vi "Configure Joystick Axis Translation.vi"(5 "Speed Profile (0: no change)":u16(ring) items=["no change", "linear", "squared", "cubed"], 6 "Axis Direction (0: no change)":u16(ring) items=["no change", "default direction", "inverted"], 7 "Maximum Speed (0)":u32, 8 "error in (no error)":errorcluster, 9 "Joystick Device Number":string, 10 "Joystick Axis Number (1)":i32=1 min=1 step=1, 11 "VISA resource name":refnum<visa-resource-name>) -> (0 "error out":errorcluster, 3 "VISA resource name out":refnum<visa-resource-name>)   [LabVIEW 2015, in "Zaber A Series.lvlib"]
doc: "Use this VI to configure the control behavior of one axis of a joystick device. \n\nEnter the device number of the joystick to be configured and select an axis to configure - 1 is the horizontal axis, 2 the vertical, and 3 is the rotation of the knob on the end of the stick. \n\nThe Maximum Speed input sets the highest velocity that will be sent to the axis the joystick controls.\n\nThe Speed Profile input controls the curve by which joystick positions are translated into velocity data.\n\nThe Axis Direction input controls whether positive joystick deflection becomes positive or negative velocity.\n\nThis VI requires that the serial port has already been opened."
uses:
  Zaber A Series.lvlib
  Private/All Commands.ctl
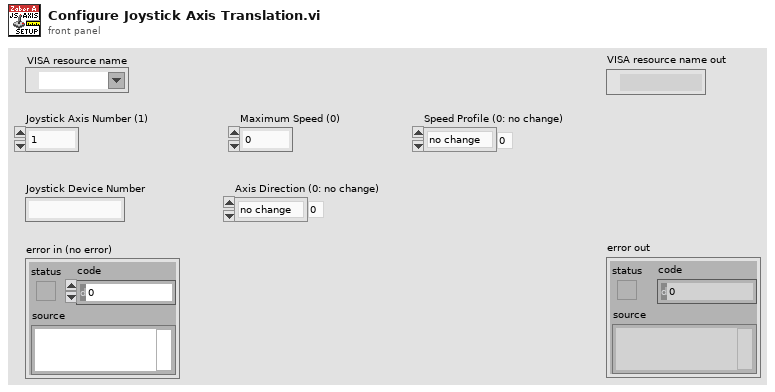
[diagram p1: front panel]
types:
  T1 = typedef "Zaber A Series.lvlib/All Commands.ctl" = string
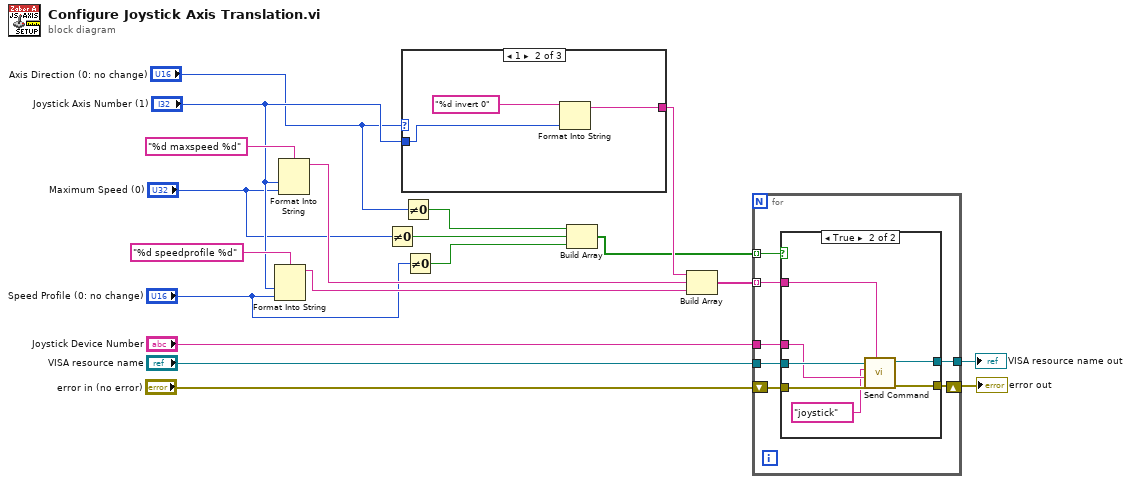
[diagram p0: block diagram]
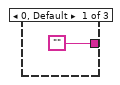
[diagram p3: hidden frame]
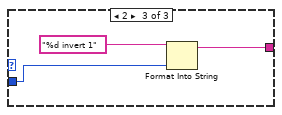
[diagram p4: hidden frame]
diagram:
  n1 = Format Into String(format string="%d speedprofile %d", "Joystick Axis Number (1)", "Speed Profile (0: no change)") -> (resulting string=w13:string)  [unwired: 2 in, 1 out]
  n2 = Format Into String(format string="%d maxspeed %d", "Joystick Axis Number (1)", "Maximum Speed (0)") -> (resulting string=w9:string)  [unwired: 2 in, 1 out]
  n3 = Not Equal To 0?(x="Maximum Speed (0)") -> (x != 0?=w11:bool)
  n4 = case shown="1" "Axis Direction (0: no change)" {
    tunnel: ["" w22 w25] -> w14
    tunnel: "Joystick Axis Number (1)" -> [_ w21 w24]
    frame 0, Default {
    }
    frame 1 {
      n5 = Format Into String(format string="%d invert 0", w21) -> (resulting string=w22:string)  [unwired: 2 in, 1 out]
    }
    frame 2 {
      n6 = Format Into String(format string="%d invert 1", w24) -> (resulting string=w25:string)  [unwired: 2 in, 1 out]
    }
  }
  n7 = Not Equal To 0?(x="Axis Direction (0: no change)") -> (x != 0?=w10:bool)
  n8 = Not Equal To 0?(x="Speed Profile (0: no change)") -> (x != 0?=w15:bool)
  n9 = Build Array(w10, w11, w15) -> (w5:bool[])
  n10 = Build Array(w14, w9, w13) -> (w4:string[])
  n11 = for {
    tunnel: [w33] -> w17
    tunnel: w5 -> [w31] mode=indexing
    tunnel: w4 -> [w30] mode=indexing
    tunnel: "VISA resource name" -> [w29]
    tunnel: "Joystick Device Number" -> [w27]
    shift-right: [w32] -> w16
    shift-left: "error in (no error)" -> [w28]
    n12 = case shown="True" w31 {
      tunnel: [w35 w42] -> w33
      tunnel: [w34 w41] -> w32
      tunnel: w30 -> [_ w40]
      tunnel: w29 -> [w35 w39]
      tunnel: w28 -> [w34 w38]
      tunnel: w27 -> [_ w37]
      frame False {
      }
      frame True {
        n13 = call "Send Command.vi"("Data"=w40, "error in (no error)"=w38, "Device and Axis"=w37, "Command"=T1 "joystick" ("Complete Command List"), "VISA resource name"=w39) -> ("error out"=w41:errorcluster, "VISA resource name out"=w42:refnum<visa-resource-name>)  [unwired: 1 in, 4 out]
      }
    }
  }
  "VISA resource name out" <- w17
  "error out" <- w16
